vi "Get Wire Type.vi"(8 "error in (no error)":errorcluster, 11 "sfixed32 in":refnum<class "sfixed32.lvclass">) -> (0 "error out":errorcluster, 2 "Wire Type":T1, 3 "sfixed32 out":refnum<class "sfixed32.lvclass">)   [LabVIEW 2020, in "Protobuf RAW.lvlib" / "sfixed32.lvclass"]
uses:
  sfixed32.lvclass
  Type Serializer/Wire Type.ctl
  sfixed32.lvclass/sfixed32.ctl
  Wire Type Group/Wire Type Group.lvclass
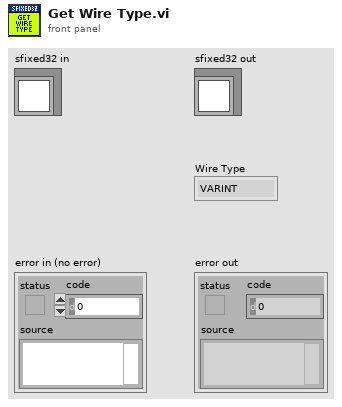
[diagram p1: front panel]
types:
  T1 = typedef "Protobuf RAW.lvlib/Wire Type Group.lvclass/Wire Type.ctl" = enum16{"VARINT", "I64", "LEN", "SGROUP", "EGROUP", "I32"}
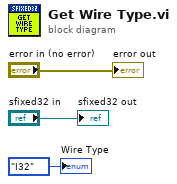
[diagram p0: block diagram]
diagram:
  "error out" <- "error in (no error)"
  "sfixed32 out" <- "sfixed32 in"
  "Wire Type" <- Wire_Type."I32" ("Wire Type")
